vi "Excel_Get_Reference_From_Range.vi"(0 "range in":refnum<k7>, 1 "error in (no error)":errorcluster) -> (2 "range out":refnum<k7>, 3 "reference":string, 4 "error out":errorcluster)   [LabVIEW 2010, in "NI_ReportGenerationToolkit.lvlib"]
uses:
  <vilib>/addons/_office/NI_ReportGenerationToolkit.lvlib
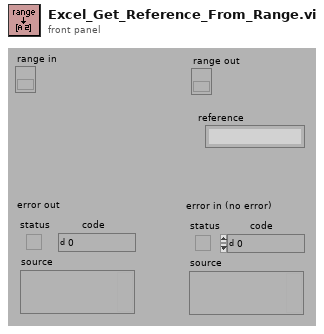
[diagram p1: front panel]
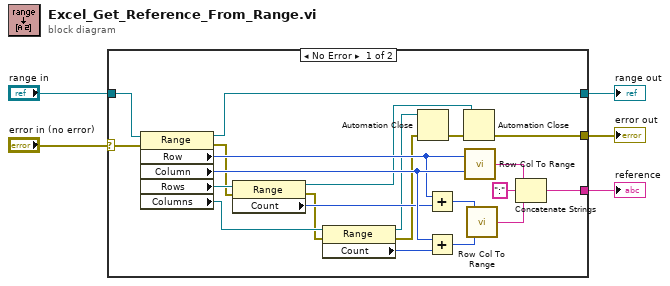
[diagram p0: block diagram]
diagram:
  n1 = case shown="No Error" "error in (no error)" {
    selector: "error in (no error)" -> [w6 w29]
    tunnel: [w27 _] -> w5
    tunnel: [w23 w28] -> w4
    tunnel: "range in" -> [w14 w28]
    tunnel: [w9 w29] -> w2
    frame No Error {
      n2 = property class="Range"(reference=w14, error in=w6) -> (reference out=w23:refnum<k7>, error out=w13:errorcluster, "Row"=w18:i32, "Column"=w20:i32, "Rows"=w15:refnum<k7>, "Columns"=w16:refnum<k7>)
      n3 = property class="Range"(reference=w15, error in=w13) -> (reference out=w8:refnum<k7>, error out=w12:errorcluster, "Count"=w17:i32)
      n4 = property class="Range"(reference=w16, error in=w12) -> (reference out=w7:refnum<k7>, error out=w11:errorcluster, "Count"=w19:i32)
      n5 = Automation Close(3:w11, 5:w7) -> (0:w10:errorcluster)
      n6 = Add(x=w18, y=w17) -> (x+y=w21:i32)
      n7 = Add(x=w20, y=w19) -> (x+y=w22:i32)
      n8 = Automation Close(3:w10, 5:w8) -> (0:w9:errorcluster)
      n9 = call <vilib>:"Row Col To Range.vi"("Column"=w20, "Row"=w18) -> ("Output String"=w24:string)
      n10 = call <vilib>:"Row Col To Range.vi"("Column"=w22, "Row"=w21) -> ("Output String"=w25:string)
      n11 = Concatenate Strings(w24, ":" ("Substring"), w25) -> (w27:string)
    }
    frame Error {
    }
  }
  "reference" <- w5
  "error out" <- w2
  "range out" <- w4
